vi "Champ-vs-foyer.vi"(2 "Compensation?":bool, 3 "Télescope Focus":dbl) -> (0 "Arcmin/pulse":dbl, 1 "Grandeur du champ":dbl)   [LabVIEW 2011]
panel:
  in  "Champ par défaut ...":dbl
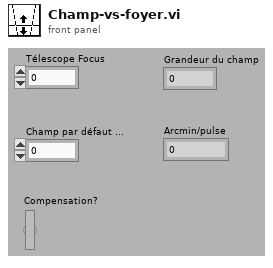
[diagram p1: front panel]
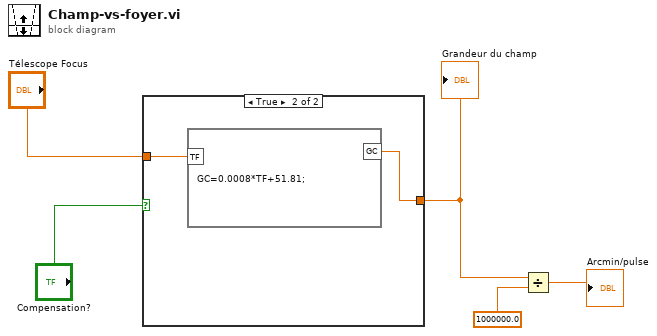
[diagram p0: block diagram]
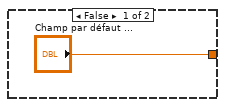
[diagram p2: hidden frame]
diagram:
  n1 = case shown="True" "Compensation?" {
    tunnel: ["Champ par défaut ..." w7] -> w3
    tunnel: "Télescope Focus" -> [_ w8]
    frame False {
    }
    frame True {
      n2 = formula code="GC=0.0008*TF+51.81;"("TF"=w8) -> ("GC"=w7:dbl)
    }
  }
  "Grandeur du champ" <- w3
  n3 = Divide(x=w3, y=1000000.0) -> (x/y=→"Arcmin/pulse":dbl)
